vi "任意角度矩形框尺寸计算及提取顶点坐标_子VI.vi"(9 "Y向图像分辨率":dbl, 10 "X向图像分辨率":dbl, 11 "ROI Descriptor(任意角度矩形)":T2 {"Contours"."Type" items=["No Selection", "Point", "Line", "Rectangle", "Oval", "Polygon", "Freehand Region", "Annulus", "Unused2", "Unused3", "Broken Line", "Freehand Line", "Rotated Rectangle"]}) -> (0 "标准矩形框坐标（L、T、R、B）":i32[](array[numeric]), 1 "矩形宽（mm）":dbl format="%#.2g", 2 "矩形长（mm）":dbl format="%#.2g", 3 "矩形框各顶点坐标值":T1, 4 "已排序的数组（X坐标）":i32[](array[numeric]), 6 "已排序的数组（Y坐标）":i32[](array[numeric]))   [LabVIEW 2018]
panel:
  # "X"
  # "（L，T）"
  # "标准矩形"
  # "任意角度矩形"
  # "(R，B)"
  # "Y"
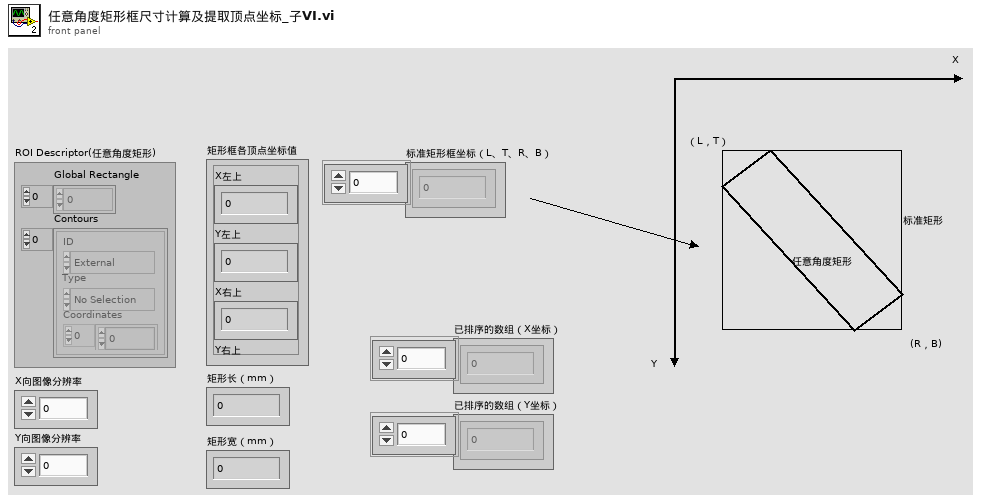
[diagram p1: front panel]
types:
  T1 = cluster{"X左上":i32, "Y左上":i32, "X右上":i32, "Y右上":i32, "X左下":i32, "Y左下":i32, "X右下":i32, "Y右下":i32}
  T2 = typedef "ROI Descriptor" = cluster{"Global Rectangle":i32[], "Contours":cluster{"ID":enum32{"External", "Internal"}, "Type":u32, "Coordinates":i32[]}[]}
  T3 = cluster{"ID":enum32{"External", "Internal"}, "Type":u32, "Coordinates":i32[]}[]
  T4 = cluster{"ID":enum32{"External", "Internal"}, "Type":u32, "Coordinates":i32[]}
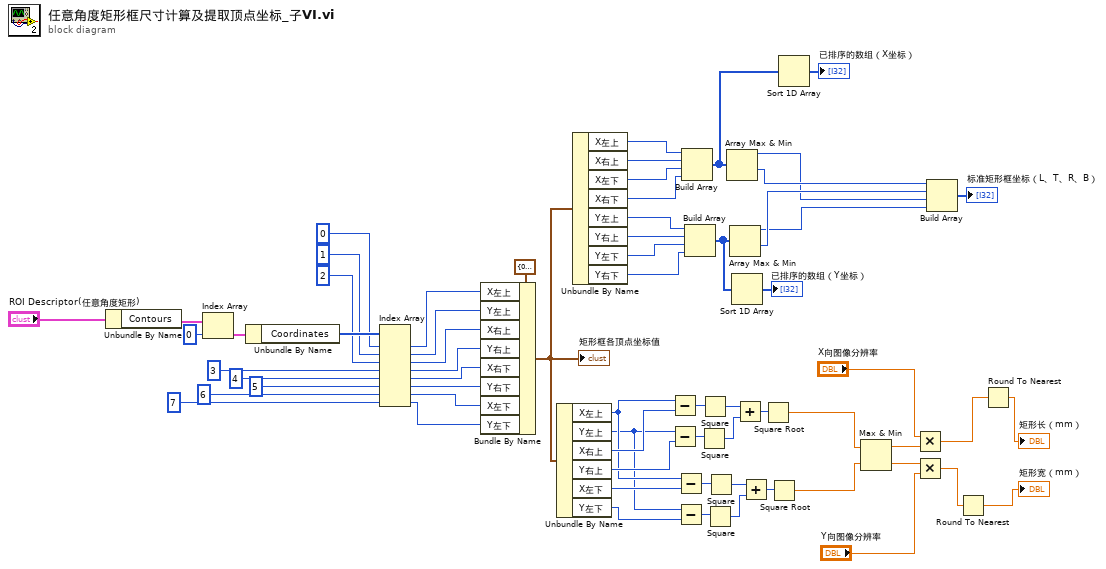
[diagram p0: block diagram]
diagram:
  n1 = Unbundle By Name("ROI Descriptor(任意角度矩形)") -> ("Contours"=w65:T3)
  n2 = Index Array(array=w65, index=0 ("索引")) -> (element=w63:T4)
  n3 = Unbundle By Name(w63) -> ("Coordinates"=w62:i32[])
  n4 = Index Array(array=w62, index #1=0 ("索引"), index #2=1 ("索引"), index #3=2 ("索引"), index #4=3 ("索引"), index #5=4 ("索引"), index #6=5 ("索引"), index #7=6 ("索引"), index #8=7 ("索引")) -> (element #1=w52:i32, element #2=w51:i32, element #3=w50:i32, element #4=w49:i32, element #5=w48:i32, element #6=w47:i32, element #7=w46:i32, element #8=w45:i32)
  n5 = Bundle By Name(cluster=T1 {"X左上"=0, "Y左上"=0, "X右上"=0, "Y右上"=0, "X左下"=0, "Y左下"=0, "X右下"=0, "Y右下"=0}, "X左上"=w52, "Y左上"=w51, "X右上"=w50, "Y右上"=w49, "X右下"=w48, "Y右下"=w47, "X左下"=w46, "Y左下"=w45) -> (w13:T1)
  "矩形框各顶点坐标值" <- w13
  n6 = Unbundle By Name(w13) -> ("X左上"=w32:i32, "Y左上"=w30:i32, "X右上"=w44:i32, "Y右上"=w41:i32, "X左下"=w31:i32, "Y左下"=w29:i32)
  n7 = Unbundle By Name(w13) -> ("X左上"=w22:i32, "X右上"=w21:i32, "X左下"=w20:i32, "X右下"=w19:i32, "Y左上"=w18:i32, "Y右上"=w17:i32, "Y左下"=w16:i32, "Y右下"=w15:i32)
  n8 = Subtract(x=w32, y=w44) -> (x-y=w43:i32)
  n9 = Subtract(x=w30, y=w41) -> (x-y=w40:i32)
  n10 = Subtract(x=w32, y=w31) -> (x-y=w33:i32)
  n11 = Subtract(x=w30, y=w29) -> (x-y=w35:i32)
  n12 = Build Array(w22, w21, w20, w19) -> (w8:i32[])
  n13 = Build Array(w18, w17, w16, w15) -> (w6:i32[])
  n14 = Square(x=w40) -> (x^2=w39:i32)
  n15 = Square(x=w43) -> (x^2=w42:i32)
  n16 = Square(x=w35) -> (x^2=w36:i32)
  n17 = Square(x=w33) -> (x^2=w34:i32)
  n18 = Array Max & Min(array=w8) -> (max value=w2:i32, min value=w4:i32)  [unwired: 2 out]
  n19 = Array Max & Min(array=w6) -> (max value=w1:i32, min value=w3:i32)  [unwired: 2 out]
  n20 = Sort 1D Array(array=w6) -> (sorted array=→"已排序的数组（Y坐标）":i32[])
  n21 = Add(x=w42, y=w39) -> (x+y=w38:i32)
  n22 = Add(x=w34, y=w36) -> (x+y=w37:i32)
  n23 = Square Root(x=w38) -> (sqrt(x)=w28:dbl)
  n24 = Square Root(x=w37) -> (sqrt(x)=w27:dbl)
  n25 = Sort 1D Array(array=w8) -> (sorted array=→"已排序的数组（X坐标）":i32[])
  n26 = Max & Min(x=w28, y=w27) -> (max(x,y)=w26:dbl, min(x,y)=w24:dbl)
  n27 = Multiply(x="X向图像分辨率", y=w26) -> (x*y=w12:dbl)
  n28 = Multiply(x=w24, y="Y向图像分辨率") -> (x*y=w10:dbl)
  n29 = Build Array(w4, w3, w2, w1) -> (→"标准矩形框坐标（L、T、R、B）":i32[])
  n30 = Round To Nearest(number=w10) -> (nearest integer value=→"矩形宽（mm）":dbl)
  n31 = Round To Nearest(number=w12) -> (nearest integer value=→"矩形长（mm）":dbl)
